vi "dfd_Convert Filter Coefficients to String.vi"(5 "indent order":i32, 7 "format string":string="%-+024.16e", 11 "filter coef":T1) -> (3 "xml string out":string)   [LabVIEW 2017, in "NI_DigFilter_Process.lvlib"]
uses:
  <vilib>/addons/Digital Filter Design/NI_DigFilter_Process.lvlib
  <vilib>/addons/Digital Filter Design/_Objects.llb/DFD Filter Coef.ctl
  <vilib>/addons/Digital Filter Design/_Objects.llb/DFD Filter Structure Type Selector.ctl
  <vilib>/addons/Digital Filter Design/NI_DigFilterLicensed.lvlib
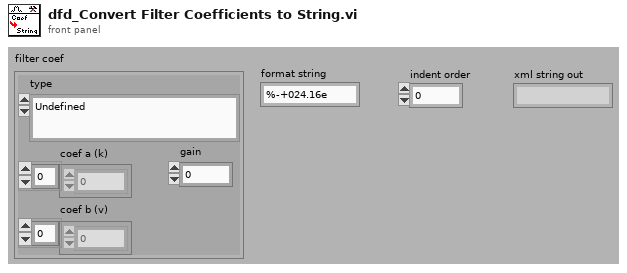
[diagram p1: front panel]
types:
  T1 = typedef "NI_DigFilterLicensed.lvlib/DFD Filter Coef.ctl" = cluster{"type":T2, "gain":dbl, "coef a (k)":dbl[], "coef b (v)":dbl[]}
  T2 = typedef "NI_DigFilterLicensed.lvlib/DFD Filter Structure Type Selector.ctl" = enum16{"Undefined", "FIR Direct Form", "FIR Direct Form Transposed", "FIR Symmetric", "FIR Antisymmetric", "IIR Direct Form I", "IIR Direct Form I Transposed", "IIR Direct Form II", "IIR Direct Form II Transposed", "IIR Cascaded Second Order Sections Form I", "IIR Cascaded Second Order Sections Form I Transposed", "IIR Cascaded Second Order Sections Form II", "IIR Cascaded Second Order Sections Form II Transposed", "Lattice Allpass (basic sections)", "Lattice Allpass (one multiplier sections)", "Lattice Allpass (normalized sections)", "Lattice AR (basic sections)", "Lattice AR (one multiplier sections)", "Lattice AR (normalized sections)", "Lattice MA (minimum phase)", "Lattice MA (maximum phase)", "Lattice ARMA (basic sections)", "Lattice ARMA (one multiplier sections)", "Lattice ARMA (normalized sections)"}
  T3 = cluster{"structure type":T2, "k":dbl[], "v":dbl[], "gain":dbl}
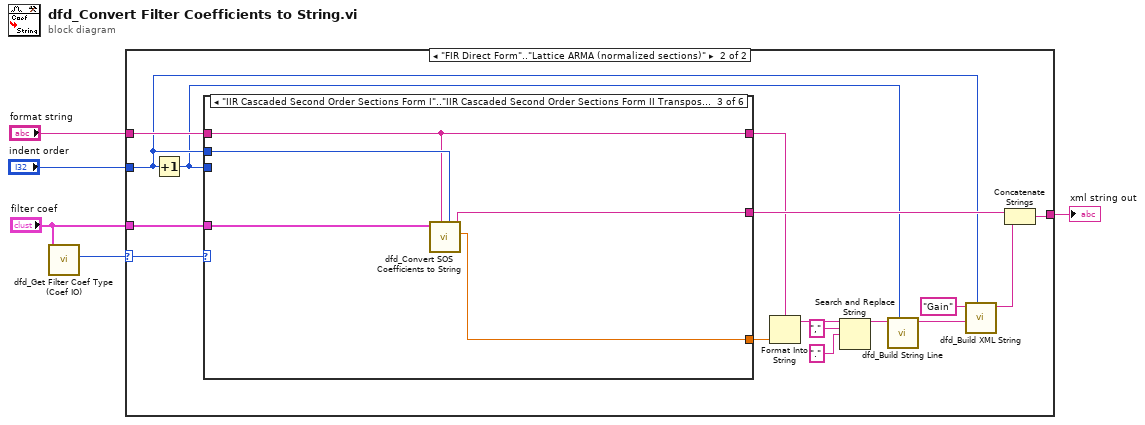
[diagram p0: block diagram]
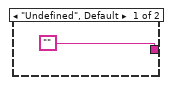
[diagram p2: hidden frame]
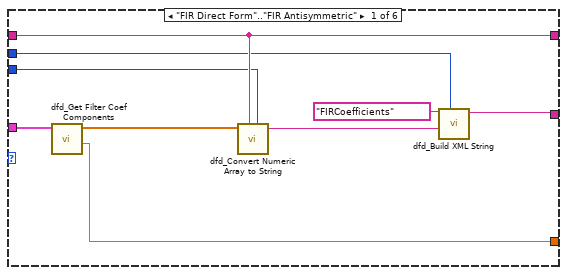
[diagram p3: hidden frame]
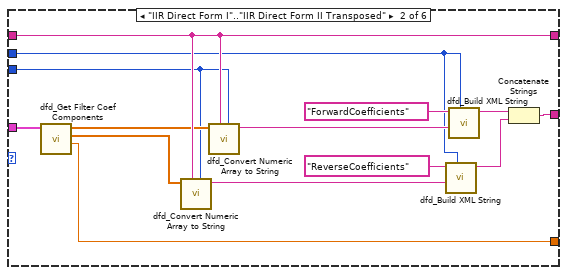
[diagram p4: hidden frame]
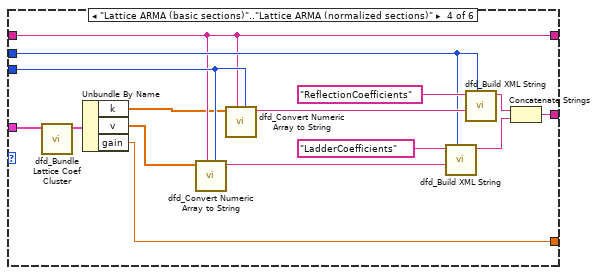
[diagram p5: hidden frame]
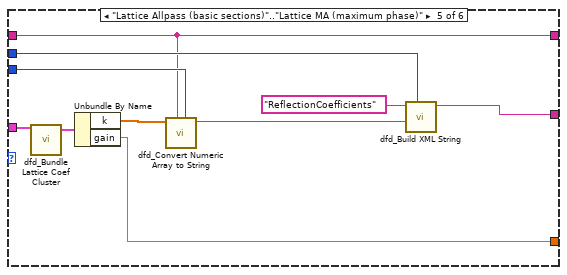
[diagram p6: hidden frame]
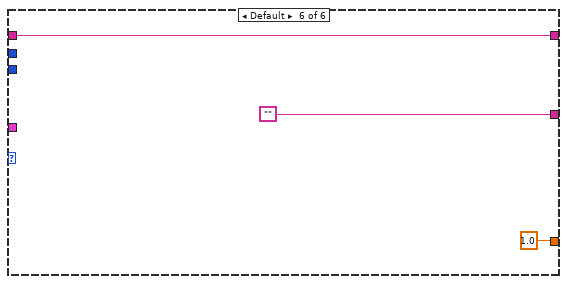
[diagram p7: hidden frame]
diagram:
  n1 = call <vilib>:"dfd_Get Filter Coef Type (Coef IO).vi"("filter coef in"="filter coef") -> ("type"=w1:T2)  [unwired: 1 in, 9 out]
  n2 = case shown="\"FIR Direct Form\"..\"Lattice ARMA (normalized sections)\"" w1 {
    selector: w1 -> [_ w14]
    tunnel: "format string" -> [_ w22]
    tunnel: ["" w18] -> w4
    tunnel: "indent order" -> [_ w16]
    tunnel: "filter coef" -> [_ w13]
    frame "Undefined", Default {
    }
    frame "FIR Direct Form".."Lattice ARMA (normalized sections)" {
      n3 = Increment(x=w16) -> (x+1=w15:i32)
      n4 = case shown="\"IIR Cascaded Second Order Sections Form I\"..\"IIR Cascaded Second Order Sections Form II Transposed\"" w14 {
        tunnel: [w29 w37 w46 w56 w70 ""] -> w20
        tunnel: w22 -> [w28 w43 w48 w57 w71 w77]
        tunnel: [w28 w43 w48 w57 w71 w77] -> w11
        tunnel: w16 -> [w27 w40 w49 w59 w73 _]
        tunnel: w15 -> [w26 w32 _ w58 w72 _]
        tunnel: [w23 w33 w47 w52 w66 1.0] -> w12
        tunnel: w13 -> [w24 w36 w50 w51 w68 _]
        frame "FIR Direct Form".."FIR Antisymmetric" {
          n5 = call <vilib>:"dfd_Get Filter Coef Components.vi"("filter coef"=w24) -> ("gain"=w23:dbl, "coef b (v)"=w25:dbl[])  [unwired: 1 in, 8 out]
          n6 = call <vilib>:"dfd_Convert Numeric Array to String.vi"("indent order"=w26, "format string"=w28, "numeric array"=w25) -> ("string"=w30:string)  [unwired: 3 in, 5 out]
          n7 = call <vilib>:"dfd_Build XML String.vi"("indent order"=w27, "string in"=w30, "element name"="FIRCoefficients") -> ("xml string out"=w29:string)  [unwired: 1 in, 7 out]
        }
        frame "IIR Direct Form I".."IIR Direct Form II Transposed" {
          n8 = call <vilib>:"dfd_Get Filter Coef Components.vi"("filter coef"=w36) -> ("gain"=w33:dbl, "coef a (k)"=w34:dbl[], "coef b (v)"=w35:dbl[])  [unwired: 1 in, 7 out]
          n9 = call <vilib>:"dfd_Convert Numeric Array to String.vi"("indent order"=w32, "format string"=w43, "numeric array"=w34) -> ("string"=w42:string)  [unwired: 3 in, 5 out]
          n10 = call <vilib>:"dfd_Convert Numeric Array to String.vi"("indent order"=w32, "format string"=w43, "numeric array"=w35) -> ("string"=w44:string)  [unwired: 3 in, 5 out]
          n11 = call <vilib>:"dfd_Build XML String.vi"("indent order"=w40, "string in"=w42, "element name"="ReverseCoefficients") -> ("xml string out"=w38:string)  [unwired: 1 in, 7 out]
          n12 = call <vilib>:"dfd_Build XML String.vi"("indent order"=w40, "string in"=w44, "element name"="ForwardCoefficients") -> ("xml string out"=w39:string)  [unwired: 1 in, 7 out]
          n13 = Concatenate Strings(w39, w38) -> (w37:string)
        }
        frame "IIR Cascaded Second Order Sections Form I".."IIR Cascaded Second Order Sections Form II Transposed" {
          n14 = call <vilib>:"dfd_Convert SOS Coefficients to String.vi"("indent order"=w49, "format string"=w48, "filter coef"=w50) -> ("gain"=w47:dbl, "XML string out"=w46:string)  [unwired: 7 out]
        }
        frame "Lattice ARMA (basic sections)".."Lattice ARMA (normalized sections)" {
          n15 = call <vilib>:"dfd_Bundle Lattice Coef Cluster.vi"("filter coef"=w51) -> ("lattice coef"=w55:T3)  [unwired: 2 in, 8 out]
          n16 = Unbundle By Name(w55) -> ("k"=w54:dbl[], "v"=w53:dbl[], "gain"=w52:dbl)
          n17 = call <vilib>:"dfd_Convert Numeric Array to String.vi"("indent order"=w58, "format string"=w57, "numeric array"=w53) -> ("string"=w63:string)  [unwired: 3 in, 5 out]
          n18 = call <vilib>:"dfd_Convert Numeric Array to String.vi"("indent order"=w58, "format string"=w57, "numeric array"=w54) -> ("string"=w64:string)  [unwired: 3 in, 5 out]
          n19 = call <vilib>:"dfd_Build XML String.vi"("indent order"=w59, "string in"=w63, "element name"="LadderCoefficients") -> ("xml string out"=w60:string)  [unwired: 1 in, 7 out]
          n20 = call <vilib>:"dfd_Build XML String.vi"("indent order"=w59, "string in"=w64, "element name"="ReflectionCoefficients") -> ("xml string out"=w61:string)  [unwired: 1 in, 7 out]
          n21 = Concatenate Strings(w61, w60) -> (w56:string)
        }
        frame "Lattice Allpass (basic sections)".."Lattice MA (maximum phase)" {
          n22 = call <vilib>:"dfd_Bundle Lattice Coef Cluster.vi"("filter coef"=w68) -> ("lattice coef"=w69:T3)  [unwired: 2 in, 8 out]
          n23 = Unbundle By Name(w69) -> ("k"=w67:dbl[], "gain"=w66:dbl)
          n24 = call <vilib>:"dfd_Convert Numeric Array to String.vi"("indent order"=w72, "format string"=w71, "numeric array"=w67) -> ("string"=w75:string)  [unwired: 1 in, 7 out]
          n25 = call <vilib>:"dfd_Build XML String.vi"("indent order"=w73, "string in"=w75, "element name"="ReflectionCoefficients") -> ("xml string out"=w70:string)  [unwired: 1 in, 7 out]
        }
        frame Default {
        }
      }
      n26 = Format Into String(format string=w11, w12) -> (resulting string=w8:string)  [unwired: 2 in, 1 out]
      n27 = Search and Replace String(input string=w8, search string=",", replace string="." ("replace string (\"\")")) -> (result string=w7:string)  [unwired: 2 in, 6 out]
      n28 = call <vilib>:"dfd_Build String Line.vi"("indent order"=w15, "string"=w7) -> ("string line"=w17:string)  [unwired: 9 out]
      n29 = call <vilib>:"dfd_Build XML String.vi"("indent order"=w16, "string in"=w17, "element name"="Gain") -> ("xml string out"=w19:string)  [unwired: 1 in, 7 out]
      n30 = Concatenate Strings(w20, w19) -> (w18:string)
    }
  }
  "xml string out" <- w4
